vi "DBC Parser File.vi"(10 "pDBCFileName":string, 11 "DevHandle":i32) -> (2 "pDBCFileName out":string, 3 "function return":u64)   [LabVIEW 2010, in "dbc_parser.lvlib"]
doc: "long long WINAPI DBC_ParserFile(int DevHandle, char* pDBCFileName);"
uses:
  dbc_parser.lvlib
  USB2XXX/trunk/USB2XXX/USB2XXX/vs2019/Release/USB2XXX.dll
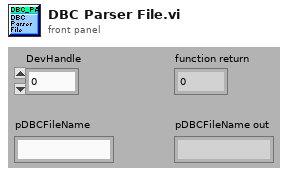
[diagram p1: front panel]
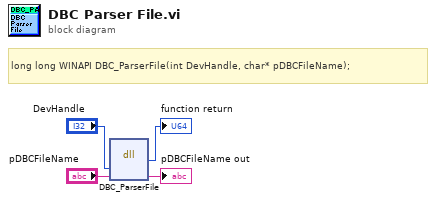
[diagram p0: block diagram]
diagram:
  # "long long WINAPI DBC_ParserFile(int DevHandle, char* pDBCFileName);"
  n1 = dll-call lib="E:/Projects/USB2XXX/trunk/USB2XXX/USB2XXX/vs2019/Release/USB2XXX.*" fn="DBC_ParserFile"("DevHandle"="DevHandle", "pDBCFileName"="pDBCFileName") -> (→"function return":u64, "pDBCFileName"=→"pDBCFileName out":string)  [unwired: 4 in, 2 out]
